vi "Tosca-Get TTL Properties.vi"(0 "State":refnum<class "State.lvclass">) -> (4 "chans":string[](array[string]), 8 "appended array":cluster{string[]}[](array[cluster]))   [LabVIEW 2020]
uses:
  Classes/State/State.lvclass
  Classes/State/State.lvclass/State.ctl
  Classes/Timeout/Timeout.lvclass/Timeout.ctl
  TTL VIs/Control Classes/Base Class/TTLController.lvclass/TTLController.ctl
  Classes/Termination/Termination.lvclass/Termination.ctl
  TTL VIs/Control Classes/Base Class/Read Name.vi
  Classes/Termination/Read Source.vi
  Classes/Termination/Read TTL.vi
  Classes/Timeout/Read TTL.vi
  Classes/State/Read Term.vi
  Classes/State/Read Timeouts.vi
  TTL VIs/Control Classes/Base Class/TTLController.lvclass
  D:/Development/epl-vi-lib/Koop/KObject Class/KObject.lvclass
  Classes/Timeout/Timeout.lvclass
  Classes/Termination/Termination.lvclass
  epl-vi-lib/Koop/KObject Class/KObject.lvclass
panel:
  out "params":string[](array[string])
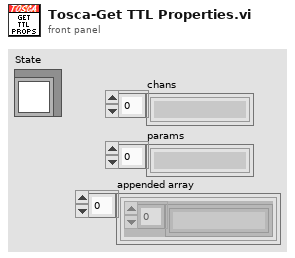
[diagram p1: front panel]
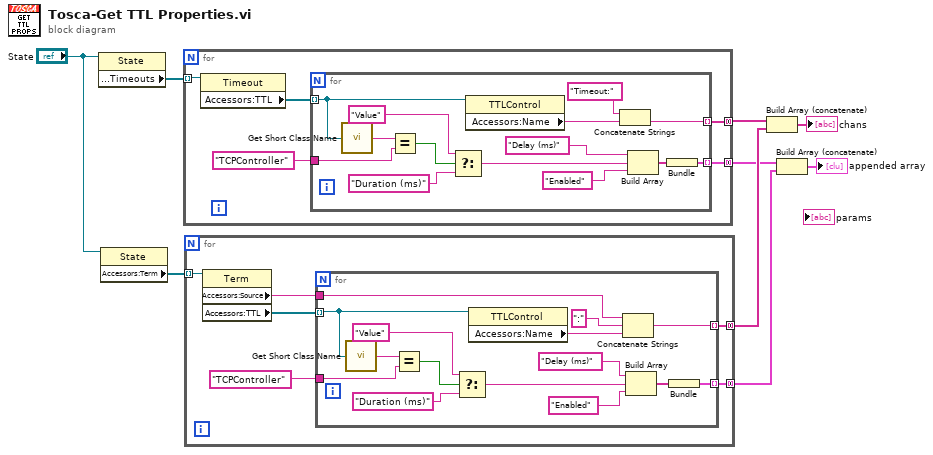
[diagram p0: block diagram]
diagram:
  n1 = property class="State"(reference="State") -> ("Accessors:Timeouts"=w3:refnum<class "Timeout.lvclass">[])  [unwired: 1 in, 2 out]
  n2 = property class="State"(reference="State") -> ("Accessors:Term"=w1:refnum<class "Termination.lvclass">[])  [unwired: 1 in, 2 out]
  n3 = for {
    tunnel: w3 -> [w12] mode=indexing
    tunnel: [w14] -> w9 mode=concatenating
    tunnel: [w13] -> w6 mode=concatenating
    n4 = property class="Timeout"(reference=w12) -> ("Accessors:TTL"=w11:refnum<class "TTLController.lvclass">[])  [unwired: 1 in, 2 out]
    n5 = for {
      tunnel: w11 -> [w21] mode=indexing
      tunnel: [w27] -> w14 mode=indexing
      tunnel: [w23] -> w13 mode=indexing
      tunnel: "TCPController" -> [w19]
      n6 = call "Get Short Class Name.vi"("KObject in"=w21) -> ("Class"=w20:string)  [unwired: 4 in]
      n7 = Equal?(x=w20, y=w19) -> (x = y?=w18:bool)
      n8 = Select(t="Value", s=w18, f="Duration (ms)") -> (s? t:f=w16:string)
      n9 = property class="TTLControl"(reference=w21) -> ("Accessors:Name"=w28:string)  [unwired: 1 in, 2 out]
      n10 = Concatenate Strings("Timeout:", w28) -> (w27:string)
      n11 = Build Array("Delay (ms)", w16, "Enabled" ("element")) -> (w24:string[])
      n12 = Bundle(w24) -> (w23:cluster{string[]})  [unwired: 1 in]
    }
  }
  n13 = for {
    tunnel: w1 -> [w32] mode=indexing
    tunnel: [w34] -> w8 mode=concatenating
    tunnel: [w33] -> w5 mode=concatenating
    n14 = property class="Term"(reference=w32) -> ("Accessors:Source"=w30:string, "Accessors:TTL"=w31:refnum<class "TTLController.lvclass">[])  [unwired: 1 in, 2 out]
    n15 = for {
      tunnel: w31 -> [w37] mode=indexing
      tunnel: [w48] -> w34 mode=indexing
      tunnel: w30 -> [w46]
      tunnel: [w43] -> w33 mode=indexing
      tunnel: "TCPController" -> [w35]
      n16 = call "Get Short Class Name.vi"("KObject in"=w37) -> ("Class"=w41:string)  [unwired: 4 in]
      n17 = Equal?(x=w41, y=w35) -> (x = y?=w40:bool)
      n18 = Select(t="Value", s=w40, f="Duration (ms)") -> (s? t:f=w36:string)
      n19 = property class="TTLControl"(reference=w37) -> ("Accessors:Name"=w49:string)  [unwired: 1 in, 2 out]
      n20 = Concatenate Strings(w46, ":", w49) -> (w48:string)
      n21 = Build Array("Delay (ms)", w36, "Enabled" ("element")) -> (w44:string[])
      n22 = Bundle(w44) -> (w43:cluster{string[]})  [unwired: 1 in]
    }
  }
  n23 = Build Array (concatenate)(w9, w8) -> (→"chans":string[])
  n24 = Build Array (concatenate)(w6, w5) -> (→"appended array":cluster{string[]}[])
